vi "LIDAR V3 FPGA Main.vi"() -> ()   [LabVIEW 2013]
uses:
  Controls/FPGA Nain State.ctl
  Controls/Scan Format Typedaf.ctl
  <vilib>/Platform/TimedLoop/XDataNode/timing_clust.ctl
  <vilib>/Platform/TimedLoop/XDataNode/nitl_modes.ctl
  <vilib>/Platform/TimedLoop/XDataNode/wakeup.ctl
  Controls/Algorithm State.ctl
  <vilib>/rvi/Emulation/niFpgaSctlEmulationGetInTimedLoop.vi
  <vilib>/rvi/Emulation/niFpgaEmulationReportErrorSimple.vi
  <vilib>/rvi/Emulation/niFpgaGetClockAttributes.vi
  <vilib>/rvi/Emulation/niFpgaCriticalErrorInLSC.vi
  <vilib>/rvi/eio/common/nirviEmuTemplateMethod_errors.vi
  <vilib>/rvi/FIFO/Fifo_Resource/nirvififoEmulationWriteFpgaImpl.vi
  <vilib>/rvi/DataTransferAndStorage/Container/Common/niFpgaContainerGetUniqueNameForEmu.vi
  <vilib>/rvi/FIFO/Fifo_Resource/nirvififoEmulationReadFpgaImpl.vi
  LIDAR V2 Globals.vi
  <vilib>/rvi/Emulation/niFpgaProcessEmulError.vi
  <vilib>/rvi/interface/RandomDataEmulation/nirviRandomDataFPGAFIFO.vi
  <vilib>/rvi/interface/RandomDataEmulation/niFpgaRandomDataHandleErrors.vi
  <vilib>/Platform/TimedLoop/XDataNode/XDataNode.xnode
  <vilib>/eio/EIONode/EIONode.xnode
  <vilib>/rvi/DataTransferAndStorage/Container/XNode/niFpgaContainer.xnode
  <vilib>/rvi/FIFO/Fifo_Resource/nirvififoEmulationWrite.vi
  <vilib>/rvi/FIFO/Fifo_Resource/nirvififoEmulationRead.vi
  <vilib>/rvi/interface/RandomDataEmulation/nirviRandomDataFpgaReadWriteTemplate.vi
  <vilib>/Platform/TimedLoop/XDataNode/XDNodeRunTimeDep.lvlib
panel:
  in  "MemDebStart":u32
  in  "MemDebEnd":u32
  in  "ReadMemSel":bool
  in  "ReadMem":bool
  in  "NextLedEn":bool
  out "SimCoarsMaxIndex":u16
  out "SimFineMaxIndex":u16
  out "AI":i16
  in  "PulseUpClck":u16=3
  in  "PulseWaitClck":u16=40
  in  "GenPulse":bool
  out "SimOut":i16
  out "SPI Idle":bool
  out "PLL Locked":bool
  in  "Clock":u8=1
  out "PLL Counter":i32
  in  "IO Module\\Apply Settings":bool
  out "LedAddress":u16
  in  "SingleCycle":bool
  in  "PulsePerLed":i16=199
  in  "ScanFormat":T1=enum."FullScanPerLed"
  in  "SamplingEnable":bool
  out "MainState":T2
  out "10thIndex":u8
  out "PulseIndex":i16
  in  "MemSel":bool
  in  "ActiveLedIndex":u16
  out "InitMem":bool
  out "PulseEnd":bool
  in  "SampPerPulse":u16=99
  out "IterReset":u16 format="%.0b"
  in  "EnAI":bool
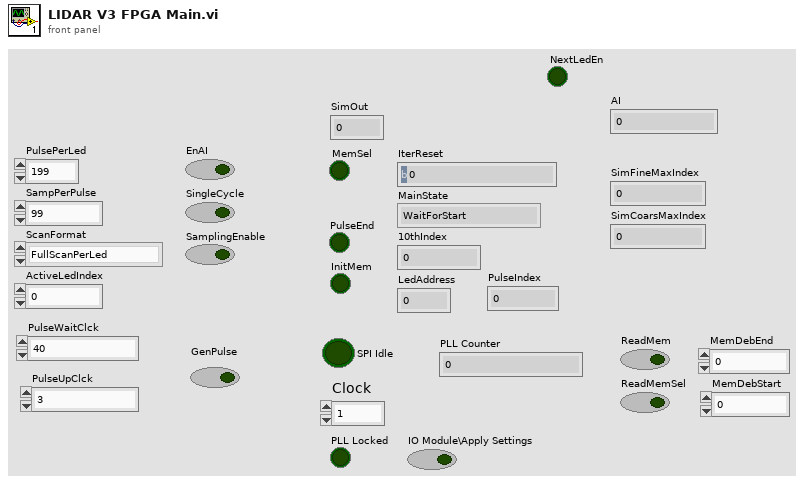
[diagram p1: front panel]
types:
  T1 = typedef "Scan Format Typedaf.ctl" = enum16{"1PulsePerLed", "FullScanPerLed"}
  T2 = typedef "FPGA Nain State.ctl" = enum16{"WaitForStart", "SetProcParams", "SelectActiveLed", "ActivatePulse", "WaitForPulseEnd", "WaitForAlgoStart", "SingleCycleEnd"}
  T3 = typedef "XDNodeRunTimeDep.lvlib/timing_clust.ctl" = cluster{"Expected End [f-1]":u64, "Actual End [f-1]":u64, "Finished Late? [f-1]":bool, "Expected End [i-1]":u64, "Actual End [i-1]":u64, "Finished Late? [i-1]":bool, "Expected Start [i]":u64, "Actual Start [i]":u64, "Expected Start [f]":u64, "Actual Start [f]":u64, "Source Name":string, "Structure Name":string, "Period":i64, "Deadline":i64, "Offset":i64, "Start":i64, "Priority":i32, "Timeout":i32, "Mode":T4, "Wakeup Reason":T5, "Error":errorcluster, "Source Type":string, "Secondary Source Type":string, "Global End Time":u64, "Global Start Time":u64, "Frame Duration":u64, "Iteration Duration":u64, "Assigned CPU":i32, "I/O Scan Engine Mode":u32}
  T4 = typedef "XDNodeRunTimeDep.lvlib/nitl_modes.ctl" = enum32{"No Change", "Process missed periods, maintain original phase", "Discard missed periods, maintain original phase", "Process missed periods, ignore original phase", "Discard missed periods, ignore original phase"}
  T5 = typedef "XDNodeRunTimeDep.lvlib/wakeup.ctl" = enum32{"Normal", "Aborted", "Asynchronous wakeup", "Timing source error", "Timed loop error", "Timeout"}
  T6 = typedef "Algorithm State.ctl" = enum16{"WaitForStart", "GetNextSignalElement", "WaitForNextSignalElem", "MultWithSinc", "CalcMax"}
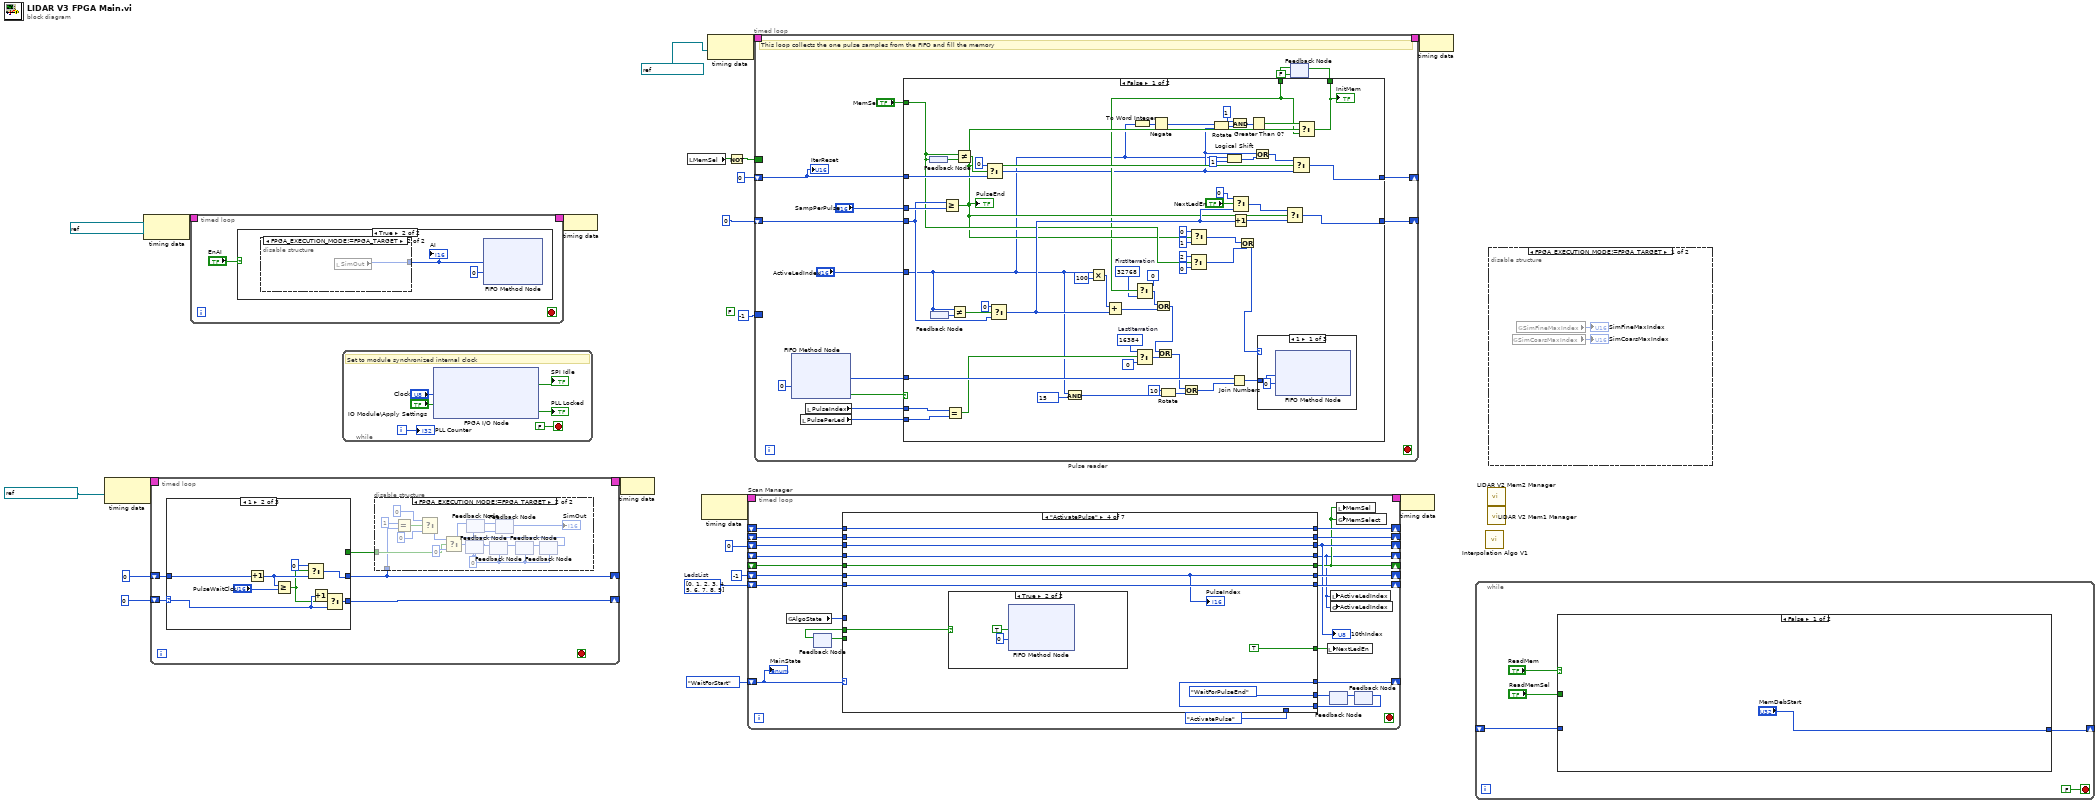
[diagram p0: block diagram]
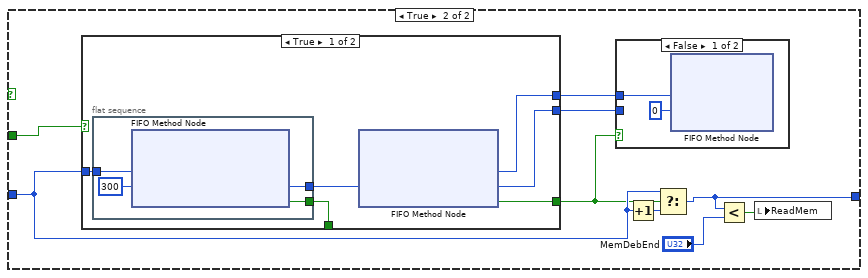
[diagram p2: hidden frame]
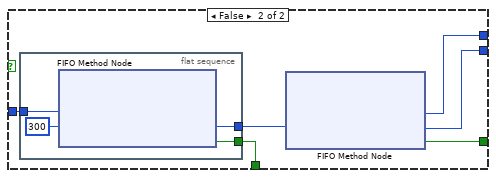
[diagram p4: hidden frame]
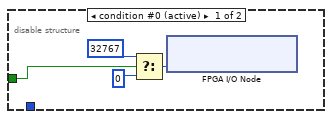
[diagram p6: hidden frame]
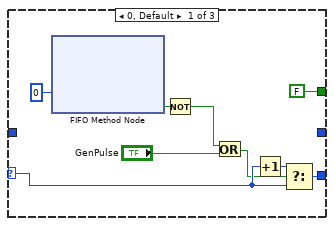
[diagram p7: hidden frame]
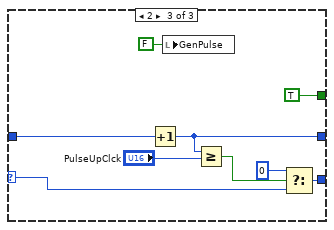
[diagram p8: hidden frame]
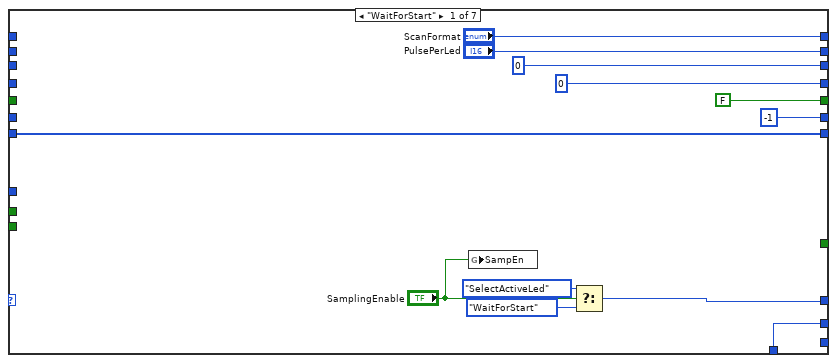
[diagram p9: hidden frame]
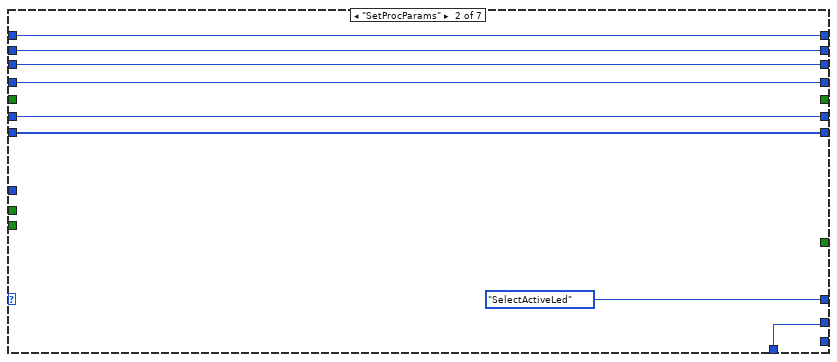
[diagram p10: hidden frame]
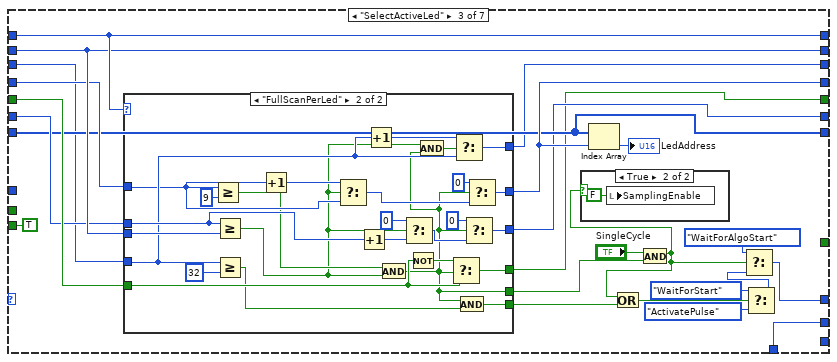
[diagram p11: hidden frame]
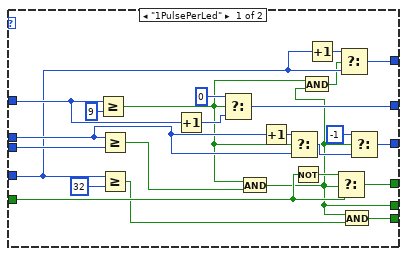
[diagram p13: hidden frame]
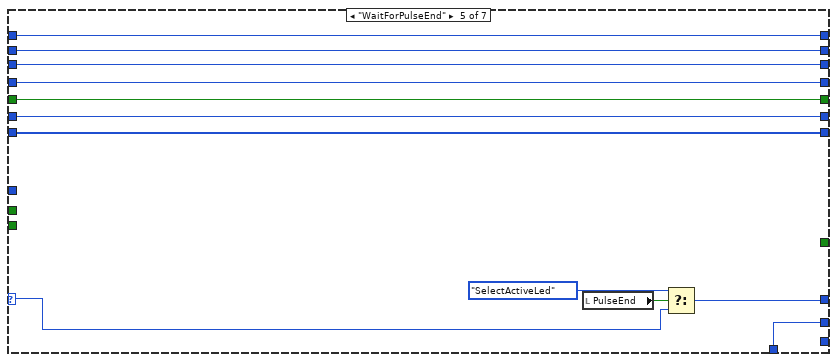
[diagram p15: hidden frame]
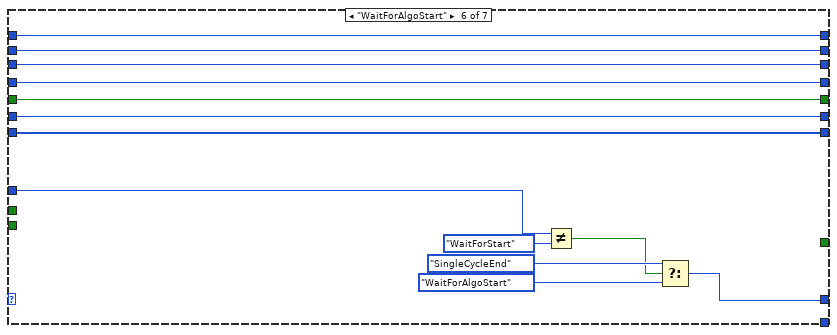
[diagram p16: hidden frame]
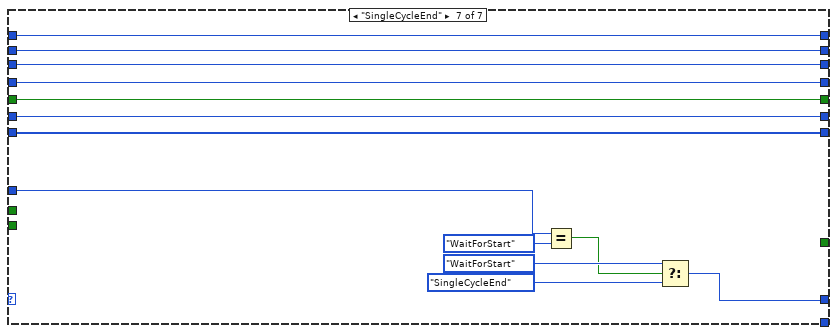
[diagram p17: hidden frame]
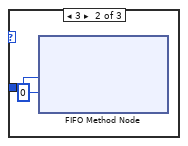
[diagram p18: hidden frame]
diagram:
  (unwired) FALSE
  w6 = u16[] [0, 1, 2, 3, 4, 5, 6, 7, 8, 9]  # LedsList
  n1 = node-c288(refnum<k21> "IO Module Clock 0" ("Source Name")) -> (w16:T3)
  n2 = node-c288(refnum<k21> "IO Module Clock 0" ("Source Name")) -> (w22:T3)
  n3 = timed-loop {
    timing: w16 -> [_]
    timing-out: [_] -> w15
    shift-right: [w26] -> _
    shift-left: i16 0 -> [w27]
    shift-right: [w23] -> _
    shift-left: u16 0 -> [w25]
    stop <- _ stop-if-true
    n4 = case shown="1" w27 {
      selector: w27 -> [w54 w62 w69]
      tunnel: [w55 w63 w70] -> w26
      tunnel: w25 -> [_ w65 w74]
      tunnel: [_ w59 w73] -> w23
      tunnel: [FALSE _ TRUE] -> w24
      frame 0, Default {
        n5 = xnode ("FIFO Method Node")("Timeout"=0) -> ("Timed Out?"=w50:bool)  [unwired: 1 in, 2 out]
        n6 = Not(x=w50) -> (.not. x?=w49:bool)
        n7 = Or(x=w49, y="GenPulse") -> (x .or. y?=w51:bool)
        n8 = Increment(x=w54) -> (x+1=w53:i16)
        n9 = Select(t=w53, s=w51, f=w54) -> (s? t:f=w55:i16)
      }
      frame 1 {
        n10 = Increment(x=w65) -> (x+1=w60:u16)
        n11 = Greater Or Equal?(x=w60, y="PulseWaitClck") -> (x >= y?=w58:bool)
        n12 = Select(t=u16 0, s=w58, f=w60) -> (s? t:f=w59:u16)
        n13 = Increment(x=w62) -> (x+1=w61:i16)
        n14 = Select(t=w61, s=w58, f=w62) -> (s? t:f=w63:i16)
      }
      frame 2 {
        n15 = Increment(x=w74) -> (x+1=w73:u16)
        n16 = local write "GenPulse"(FALSE ("GenPulse")) -> ()
        n17 = Greater Or Equal?(x=w73, y="PulseUpClck") -> (x >= y?=w71:bool)
        n18 = Select(t=i16 0, s=w71, f=w69) -> (s? t:f=w70:i16)
      }
    }
    n19 = disable-structure shown="FPGA_EXECUTION_MODE!=FPGA_TARGET" {
      disable-tunnel: w24 -> [w29 w38]
      disable-tunnel: w23 -> [_ w37]
      frame condition #0 (active) {
        n20 = Select(t=i16 32767 ("IO Module\\AO 0"), s=w29, f=i16 0 ("IO Module\\AO 0")) -> (s? t:f=w28:i16)
        n21 = xnode "FPGA I/O Node"("IO Module\\AO 0"=w28) -> ()  [unwired: 1 in, 1 out]
      }
      frame condition #1 {
        w42 = i16 0 ("IO Module\\AO 0")
        n22 = Equal?(x=u16 1, y=w37) -> (x = y?=w35:bool)
        n23 = Select(t=i16 0 ("IO Module\\AO 0"), s=w35, f=i16 0) -> (s? t:f=w36:i16)
        n24 = Select(t=w36, s=w38, f=i16 0 ("IO Module\\AO 0")) -> (s? t:f=w39:i16)
        n25 = feedback-in #1(w39) -> ()
        n26 = feedback #1(w42) -> (w47:i16)
        n27 = feedback #2(w42) -> (w43:i16)
        n28 = feedback #3(w42) -> (w46:i16)
        n29 = feedback-in #3(w47) -> ()
        n30 = feedback #4(w42) -> (→"SimOut":i16)
        n31 = feedback-in #4(w43) -> ()
        n32 = feedback #5(w42) -> (w45:i16)
        n33 = feedback-in #5(w46) -> ()
        n34 = feedback #6(w42) -> (w44:i16)
        n35 = feedback-in #2(w44) -> ()
        n36 = feedback-in #6(w45) -> ()
      }
    }
  }
  n37 = timed-loop {
    timing: w22 -> [_]
    timing-out: [_] -> w21
    stop <- _ stop-if-true
    n38 = case shown="True" "EnAI" {
      frame False {
      }
      frame True {
        n39 = disable-structure shown="FPGA_EXECUTION_MODE!=FPGA_TARGET" {
          disable-tunnel: [w80 w81] -> w78
          frame condition #0 (active) {
            n40 = xnode "FPGA I/O Node"() -> ("IO Module\\AI 0"=w80:i16)  [unwired: 1 in, 1 out]
          }
          frame condition #1 {
            n41 = local read "SimOut"() -> (w81:i16)
          }
        }
        "AI" <- w78
        n42 = xnode ("FIFO Method Node")("Element"=w78, "Timeout"=0) -> ()  [unwired: 1 in, 2 out]
      }
    }
  }
  n43 = while {
    i -> [w86]
    stop <- FALSE stop-if-true
    # "Set to module synchronized internal clock"
    n44 = xnode "FPGA I/O Node"("IO Module\\Clock Select"="Clock", "IO Module\\Apply Settings"="IO Module\\Apply Settings") -> ("IO Module\\SPI Idle"=→"SPI Idle":bool, "IO Module\\PLL Locked"=→"PLL Locked":bool)  [unwired: 4 in, 4 out]
    "PLL Counter" <- w86
  }
  n45 = node-c288(w21) -> ()
  n46 = node-c288(w15) -> ()
  n47 = local read "MemSel"() -> (w11:bool)
  n48 = node-c288() -> (w18:T3)  [unwired: 1 in]
  n49 = node-c288(refnum<k21> "100 MHz Clock" ("Source Name")) -> (w20:T3)
  n50 = Not(x=w11) -> (.not. x?=w10:bool)
  n51 = timed-loop "Scan Manager" {
    timing: w18 -> [_]
    timing-out: [_] -> w17
    shift-right: [w112] -> _
    shift-left: FPGA_Nain_State."WaitForStart" ("MainState") -> [w113]
    shift-right: [w111] -> _
    shift-left: _ -> [w109]
    shift-right: [w110] -> _
    shift-left: _ -> [w108]
    shift-right: [w101] -> _
    shift-left: u8 0 ("10thIndex") -> [w107]
    shift-right: [w91] -> _
    shift-left: _ -> [w106]
    shift-right: [w95] -> _
    shift-left: _ -> [w105]
    shift-right: [w104] -> _
    shift-left: i16 -1 -> [w94]
    shift-right: [w102] -> _
    shift-left: w6 -> [w103]
    stop <- _ stop-if-true
    n52 = global read "LIDAR V2 Globals.vi" "AlgoState"() -> (w90:T6)
    n53 = feedback #7() -> (w92:bool)  [unwired: 1 in]
    n54 = feedback #8() -> (w98:T2)  [unwired: 1 in]
    n55 = feedback #9() -> (w97:T2)  [unwired: 1 in]
    n56 = case shown="\"ActivatePulse\"" w113 {
      selector: w113 -> [_ _ _ _ w227 _ _]
      tunnel: [w123 FPGA_Nain_State."SelectActiveLed" ("MainState") w137 w211 w226 w237 w250] -> w112
      tunnel: ["ScanFormat" w129 w157 w219 w233 w246 w259] -> w111
      tunnel: ["PulsePerLed" w128 w155 w218 w232 w245 w258] -> w110
      tunnel: w109 -> [_ w129 w157 w219 w233 w246 w259]
      tunnel: w108 -> [_ w128 w155 w218 w232 w245 w258]
      tunnel: [u8 0 ("10thIndex") w127 w145 w217 w231 w244 w257] -> w101
      tunnel: w107 -> [_ w127 w146 w217 w231 w244 w257]
      tunnel: [u16 0 ("ActiveLedIndex") w126 w152 w216 w230 w243 w256] -> w91
      tunnel: w106 -> [_ w126 w153 w216 w230 w243 w256]
      tunnel: [FALSE _ w148 w215 w229 w242 w255] -> w95
      tunnel: w105 -> [_ _ w156 w215 w229 w242 w255]
      tunnel: [i16 -1 ("t") w132 w149 w209 w224 w241 w254] -> w104
      tunnel: w94 -> [_ w132 w154 w209 w224 w241 w254]
      tunnel: w103 -> [w121 w131 w151 w214 w223 w240 w253]
      tunnel: [w121 w131 w151 w214 w223 w240 w253] -> w102
      tunnel: [_ _ _ TRUE ("SampEnable") _ _ _] -> w100
      tunnel: [w120 w130 w144 FPGA_Nain_State."WaitForPulseEnd" ("MainState") w222 _ _] -> w99
      tunnel: w97 -> [_ _ _ w211 _ _ _]
      tunnel: FPGA_Nain_State."ActivatePulse" ("MainState") -> [w120 w130 w144 _ w222 _ _]
      tunnel: [_ _ TRUE _ _ _ _] -> w93
      tunnel: w92 -> [_ _ _ w210 _ _ _]
      tunnel: w90 -> [_ _ _ _ _ w234 w248]
      frame "WaitForStart" {
        n57 = global write "LIDAR V2 Globals.vi" "SampEn"("SamplingEnable") -> ()
        n58 = Select(t=FPGA_Nain_State."SelectActiveLed" ("MainState"), s="SamplingEnable", f=FPGA_Nain_State."WaitForStart" ("MainState")) -> (s? t:f=w123:T2)
      }
      frame "SetProcParams" {
      }
      frame "SelectActiveLed" {
        n59 = case shown="\"FullScanPerLed\"" w157 {
          tunnel: w156 -> [w174 w204]
          tunnel: w146 -> [w167 w199]
          tunnel: w155 -> [w177 w206]
          tunnel: w153 -> [w180 w190]
          tunnel: w154 -> [w176 w205]
          tunnel: [w168 w186] -> w152
          tunnel: [w163 w188] -> w149
          tunnel: [w171 w202] -> w148
          tunnel: [w169 w200] -> w142
          tunnel: [w165 w197] -> w145
          tunnel: [w159 w183] -> w143
          frame "1PulsePerLed" {
            n60 = Greater Or Equal?(x=w180, y=u16 9) -> (x >= y?=w161:bool)
            n61 = Greater Or Equal?(x=w176, y=w177) -> (x >= y?=w172:bool)
            n62 = Greater Or Equal?(x=w167, y=u8 32) -> (x >= y?=w170:bool)
            n63 = Increment(x=w180) -> (x+1=w179:u16)
            n64 = Select(t=u16 0, s=w161, f=w179) -> (s? t:f=w168:u16)
            n65 = And(x=w161, y=w172) -> (x .and. y?=w159:bool)
            n66 = Increment(x=w176) -> (x+1=w175:i16)
            n67 = Select(t=w175, s=w161, f=w176) -> (s? t:f=w164:i16)
            n68 = Not(x=w174) -> (.not. x?=w173:bool)
            n69 = And(x=w161, y=w159) -> (x .and. y?=w160:bool)
            n70 = Increment(x=w167) -> (x+1=w166:u8)
            n71 = Select(t=w173, s=w159, f=w174) -> (s? t:f=w171:bool)
            n72 = Select(t=w166, s=w160, f=w167) -> (s? t:f=w165:u8)
            n73 = And(x=w159, y=w170) -> (x .and. y?=w169:bool)
            n74 = Select(t=i16 -1, s=w159, f=w164) -> (s? t:f=w163:i16)
          }
          frame "FullScanPerLed" {
            n75 = Greater Or Equal?(x=w190, y=u16 9) -> (x >= y?=w189:bool)
            n76 = Greater Or Equal?(x=w205, y=w206) -> (x >= y?=w184:bool)
            n77 = Greater Or Equal?(x=w199, y=u8 32) -> (x >= y?=w201:bool)
            n78 = Increment(x=w190) -> (x+1=w191:u16)
            n79 = Select(t=w191, s=w184, f=w190) -> (s? t:f=w187:u16)
            n80 = Increment(x=w205) -> (x+1=w193:i16)
            n81 = Increment(x=w199) -> (x+1=w198:u8)
            n82 = And(x=w189, y=w184) -> (x .and. y?=w183:bool)
            n83 = Select(t=i16 0, s=w184, f=w193) -> (s? t:f=w196:i16)
            n84 = Not(x=w204) -> (.not. x?=w203:bool)
            n85 = And(x=w184, y=w183) -> (x .and. y?=w194:bool)
            n86 = Select(t=w203, s=w183, f=w204) -> (s? t:f=w202:bool)
            n87 = Select(t=w198, s=w194, f=w199) -> (s? t:f=w197:u8)
            n88 = And(x=w183, y=w201) -> (x .and. y?=w200:bool)
            n89 = Select(t=i16 0, s=w183, f=w196) -> (s? t:f=w188:i16)
            n90 = Select(t=u16 0, s=w183, f=w187) -> (s? t:f=w186:u16)
          }
        }
        n91 = Index Array(array=w151, index=w152) -> (element=→"LedAddress":u16)
        n92 = And(x="SingleCycle", y=w143) -> (x .and. y?=w134:bool)
        n93 = case shown="True" w134 {
          frame False {
          }
          frame True {
            n94 = local write "SamplingEnable"(FALSE ("SamplingEnable")) -> ()
          }
        }
        n95 = Or(x=w134, y=w142) -> (x .or. y?=w141:bool)
        n96 = Select(t=FPGA_Nain_State."WaitForStart" ("MainState"), s=w141, f=FPGA_Nain_State."ActivatePulse" ("MainState")) -> (s? t:f=w138:T2)
        n97 = Select(t=FPGA_Nain_State."WaitForAlgoStart" ("MainState"), s=w134, f=w138) -> (s? t:f=w137:T2)
      }
      frame "ActivatePulse" {
        n98 = case shown="True" w210 {
          frame False {
          }
          frame True {
            n99 = xnode ("FIFO Method Node")("Element"=TRUE ("GenPulse"), "Timeout"=0) -> ()  [unwired: 1 in, 2 out]
          }
        }
        "PulseIndex" <- w209
      }
      frame "WaitForPulseEnd" {
        n100 = local read "PulseEnd"() -> (w228:bool)
        n101 = Select(t=FPGA_Nain_State."SelectActiveLed", s=w228, f=w227) -> (s? t:f=w226:T2)
      }
      frame "WaitForAlgoStart" {
        n102 = Not Equal?(x=w234, y=Algorithm_State."WaitForStart") -> (x != y?=w235:bool)
        n103 = Select(t=FPGA_Nain_State."SingleCycleEnd", s=w235, f=FPGA_Nain_State."WaitForAlgoStart" ("MainState")) -> (s? t:f=w237:T2)
      }
      frame "SingleCycleEnd" {
        n104 = Equal?(x=w248, y=Algorithm_State."WaitForStart") -> (x = y?=w247:bool)
        n105 = Select(t=FPGA_Nain_State."WaitForStart", s=w247, f=FPGA_Nain_State."SingleCycleEnd" ("MainState")) -> (s? t:f=w250:T2)
      }
    }
    "10thIndex" <- w101
    n106 = feedback-in #7(w93) -> ()
    n107 = local write "NextLedEn"(w100) -> ()
    n108 = feedback-in #8(w99) -> ()
    n109 = local write "ActiveLedIndex"(w91) -> ()
    n110 = global write "LIDAR V2 Globals.vi" "ActiveLedIndex"(w91) -> ()
    n111 = local write "MemSel"(w95) -> ()
    n112 = global write "LIDAR V2 Globals.vi" "MemSelect"(w95) -> ()
    n113 = feedback-in #9(w98) -> ()
    "MainState" <- w113
  }
  n114 = timed-loop "Pulse reader" {
    timing: w20 -> [_]
    timing-out: [_] -> w19
    border: i16 -1 ("#Cycle") -> [_]
    shift-right: [w273] -> _
    shift-left: u16 0 -> [w271]
    border: w10 -> [_]
    shift-right: [w263] -> _
    shift-left: u16 0 -> [w262]
    stop <- _ stop-if-true
    # "This loop collects the one pulse samples from the FIFO and fill the memory"
    n115 = xnode ("FIFO Method Node")("Timeout"=0) -> ("Element"=w275:i16, "Timed Out?"=w274:bool)  [unwired: 1 in, 1 out]
    n116 = local read "PulsePerLed"() -> (w264:i16)
    n117 = local read "PulseIndex"() -> (w265:i16)
    n118 = feedback #10(FALSE) -> (w269:bool)
    n119 = case shown="False" w274 {
      tunnel: w275 -> [w330 _]
      tunnel: "ActiveLedIndex" -> [w278 _]
      tunnel: "SampPerPulse" -> [w329 _]
      tunnel: [w307 w342] -> w273
      tunnel: w271 -> [w331 w342]
      tunnel: [w284 w341] -> w270
      tunnel: w269 -> [w283 w341]
      tunnel: "MemSel" -> [w297 _]
      tunnel: w265 -> [w327 _]
      tunnel: w264 -> [w326 _]
      tunnel: [w308 w340] -> w263
      tunnel: w262 -> [w325 w340]
      frame False {
        w318 = u16 16384  # LastIterration
        w281 = u16 32768  # FirstIterration
        n120 = feedback #11() -> (w333:bool)
        n121 = feedback-in #11(w297) -> ()
        n122 = feedback #12() -> (w279:u16)
        n123 = feedback-in #12(w278) -> ()
        n124 = Greater Or Equal?(x=w325, y=w329) -> (x >= y?=w286:bool)
        "PulseEnd" <- w286
        n125 = Equal?(x=w327, y=w326) -> (x = y?=w328:bool)
        n126 = Not Equal?(x=w278, y=w279) -> (x != y?=w277:bool)
        n127 = Not Equal?(x=w297, y=w333) -> (x != y?=w334:bool)
        n128 = Select(t=u16 0, s=w334, f=w331) -> (s? t:f=w282:u16)
        n129 = Select(t=u16 0, s=w277, f=w325) -> (s? t:f=w303:u16)
        n130 = And(x=w278, y=u16 15) -> (x .and. y?=w314:u16)
        n131 = Multiply(x=w278, y=u16 100) -> (x*y=w323:u16)
        n132 = Add(x=w323, y=w303) -> (x+y=w322:u16)
        n133 = To Word Integer(number=w278) -> (16bit integer=w291:i16)
        n134 = Select(t=u16 0 ("x"), s=w283, f=w281) -> (s? t:f=w321:u16)
        n135 = Select(t=w318, s=w328, f=u16 0 ("x")) -> (s? t:f=w317:u16)
        n136 = Negate(x=w291) -> (-x=w287:i16)
        n137 = Or(x=w321, y=w322) -> (x .or. y?=w316:u16)
        n138 = Or(x=w316, y=w317) -> (x .or. y?=w311:u16)
        n139 = Rotate(1:w314, 2:i16 10 ("y")) -> (0:w312:u16)
        n140 = Or(x=w311, y=w312) -> (x .or. y?=w310:u16)
        n141 = Select(t=i16 2, s=w297, f=i16 0) -> (s? t:f=w293:i16)
        n142 = Select(t=i16 0, s=w286, f=i16 1) -> (s? t:f=w292:i16)
        n143 = Rotate(1:w282, 2:w287) -> (0:w288:u16)
        n144 = Logical Shift(y=w278, x=u16 1) -> (x << y=w302:u16)
        n145 = Join Numbers(hi=w330, lo=w310) -> ((hi.lo)=w320:u32)
        n146 = And(x=u16 1, y=w288) -> (x .and. y?=w290:u16)
        n147 = Select(t=u16 0, s="NextLedEn", f=w303) -> (s? t:f=w304:u16)
        n148 = Increment(x=w303) -> (x+1=w309:u16)
        n149 = Or(x=w292, y=w293) -> (x .or. y?=w294:i16)
        n150 = Greater Than 0?(x=w290) -> (x > 0?=w285:bool)
        n151 = Or(x=w282, y=w302) -> (x .or. y?=w300:u16)
        n152 = case shown="1" w294 {
          tunnel: w320 -> [w336 w338 _]
          frame 1 {
            n153 = xnode ("FIFO Method Node")("Element"=w336, "Timeout"=0) -> ()  [unwired: 1 in, 2 out]
          }
          frame 3 {
            n154 = xnode ("FIFO Method Node")("Element"=w338, "Timeout"=0) -> ()  [unwired: 1 in, 2 out]
          }
          frame Default {
          }
        }
        n155 = Select(t=w304, s=w286, f=w309) -> (s? t:f=w308:u16)
        n156 = Select(t=w300, s=w286, f=w282) -> (s? t:f=w307:u16)
        n157 = Select(t=w285, s=w286, f=w283) -> (s? t:f=w284:bool)
        "InitMem" <- w284
      }
      frame True {
      }
    }
    n158 = feedback-in #10(w270) -> ()
    "IterReset" <- w271
  }
  n159 = node-c288(w17) -> ()
  n160 = node-c288(w19) -> ()
  n161 = while {
    shift-right: [w347] -> _
    shift-left: _ -> [w346]
    stop <- FALSE stop-if-true
    n162 = case shown="False" "ReadMem" {
      tunnel: "ReadMemSel" -> [_ w354]
      tunnel: ["MemDebStart" w357] -> w347
      tunnel: w346 -> [_ w359]
      frame False {
      }
      frame True {
        n163 = case shown="True" w354 {
          tunnel: w359 -> [w366 w374]
          tunnel: [w365 w373] -> w351
          tunnel: [w364 w372] -> w353
          tunnel: [w363 w371] -> w352
          tunnel: [w362 w370] -> _
          frame True {
            n164 = flat-sequence {
              tunnel: w366 -> [w369]
              tunnel: [w368] -> w363
              tunnel: [w367] -> w362
              frame #0 {
                w368 = 300 ("Timeout")
                n165 = xnode ("FIFO Method Node")("Element"=w369, "Timeout"=w368) -> ("Timed Out?"=w367:bool)  [unwired: 1 in, 1 out]
              }
            }
            n166 = xnode ("FIFO Method Node")("Timeout"=w363) -> ("Element"=w364:u64, "Timed Out?"=w365:bool)  [unwired: 1 in, 1 out]
          }
          frame False {
            n167 = flat-sequence {
              tunnel: w374 -> [w377]
              tunnel: [w376] -> w371
              tunnel: [w375] -> w370
              frame #0 {
                w376 = 300 ("Timeout")
                n168 = xnode ("FIFO Method Node")("Element"=w377, "Timeout"=w376) -> ("Timed Out?"=w375:bool)  [unwired: 1 in, 1 out]
              }
            }
            n169 = xnode ("FIFO Method Node")("Timeout"=w371) -> ("Element"=w372:u64, "Timed Out?"=w373:bool)  [unwired: 1 in, 1 out]
          }
        }
        n170 = case shown="False" w351 {
          tunnel: w353 -> [w361 _]
          tunnel: w352 -> [_ _]
          frame False {
            n171 = xnode ("FIFO Method Node")("Element"=w361, "Timeout"=0) -> ()  [unwired: 1 in, 2 out]
          }
          frame True {
          }
        }
        n172 = Increment(x=w359) -> (x+1=w358:u32)
        n173 = Select(t=w359, s=w351, f=w358) -> (s? t:f=w357:u32)
        n174 = Less?(x=w357, y="MemDebEnd") -> (x < y?=w355:bool)
        n175 = local write "ReadMem"(w355) -> ()
      }
    }
  }
  n176 = call "Interpolation Algo V1.vi"() -> ()  [unwired: 10 in, 2 out]
  n177 = call "LIDAR V2 Mem2 Manager.vi"() -> ()  [unwired: 12 in]
  n178 = call "LIDAR V2 Mem1 Manager.vi"() -> ()  [unwired: 12 in]
  n179 = disable-structure shown="FPGA_EXECUTION_MODE!=FPGA_TARGET" {
    frame condition #0 {
      n180 = global read "LIDAR V2 Globals.vi" "SimCoarsMaxIndex"() -> (→"SimCoarsMaxIndex":u16)
      n181 = global read "LIDAR V2 Globals.vi" "SimFineMaxIndex"() -> (→"SimFineMaxIndex":u16)
    }
    frame condition #1 (active) {
    }
  }
